vi "Entry.vi"(8 "error in (no error)":errorcluster, 11 "New State":refnum<class "Command.lvclass">) -> (0 "error out":errorcluster, 3 "State out":refnum<class "Command.lvclass">)   [LabVIEW 2013, in "Command Processor.lvlib" / "Command.lvlib" / "Command.lvclass"]
doc: "This is an abstract method. Override this method to define the behavior when you enter the state."
uses:
  Command.lvclass
  <vilib>/ni/Actors/State Actor/State Actor/State Actor.lvclass
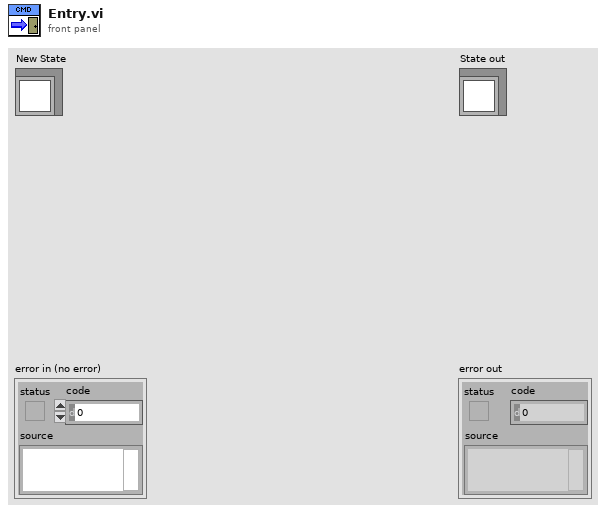
[diagram p1: front panel]
types:
  T1 = typedef "Command Processor.lvlib/Command.lvlib/Command.lvclass/Command Status.ctl" = cluster{"Command Name":string, "Current State Status":T2, "Command Start Time":timestamp, "Command End Time":timestamp, "Previous State Status":T2}
  T2 = typedef "Command Processor.lvlib/Command.lvlib/Command.lvclass/State Status.ctl" = cluster{"State Name":string, "State Entry Time":timestamp, "State Exit Time":timestamp}
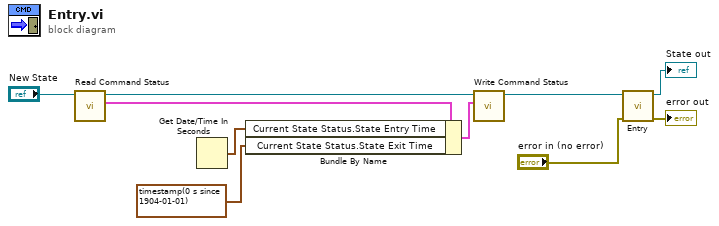
[diagram p0: block diagram]
diagram:
  n1 = call-dynamic "Read Command Status.vi"("Command in"="New State") -> ("Command Status"=w4:T1, "Command out"=w5:refnum<class "Command.lvclass">)  [unwired: 8 in, 1 out]
  n2 = Get Date/Time In Seconds() -> (seconds since 1Jan1904=w2:timestamp)
  n3 = Bundle By Name(cluster=w4, "Current State Status.State Entry Time"=w2, "Current State Status.State Exit Time"=timestamp(0 s since 1904-01-01)) -> (w3:T1)
  n4 = call-dynamic "Write Command Status.vi"("Command Status"=w3, "Command in"=w5) -> ("Command out"=w6:refnum<class "Command.lvclass">)  [unwired: 8 in, 1 out]
  n5 = call-parent "Entry.vi"("error in (no error)"="error in (no error)", "New State"=w6) -> ("error out"=→"error out":errorcluster, "State out"=→"State out":refnum<class "Command.lvclass">)  [unwired: 8 in]
